vi "sys_get dynamic system class.vi"(11 "Dynamic System":T1) -> (2 "appended path":path, 3 "Dynamic-System out":refnum<class "Dynamic-System.lvclass">)   [LabVIEW 2025]
uses:
  Classes/Dynamic-System/Dynamic-System.lvclass
  Classes/mass-spring-damper/mass-spring-damper.lvclass
  Classes/water-tank/water-tank.lvclass
  C:/Users/grove/Desktop/LabVIEW/Git/dynamic-systems/Classes/Dynamic-System/Dynamic-System.lvclass
  C:/Users/grove/Desktop/LabVIEW/Git/dynamic-systems/Classes/mass-spring-damper/mass-spring-damper.lvclass
  C:/Users/grove/Desktop/LabVIEW/Git/dynamic-systems/Classes/water-tank/water-tank.lvclass
  Classes/Dynamic-System/dynamic system selection.ctl
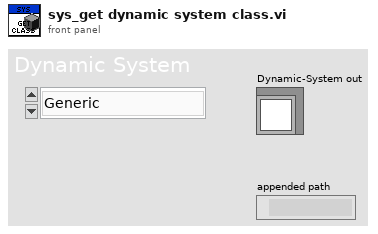
[diagram p1: front panel]
types:
  T1 = typedef "dynamic system selection.ctl" = enum16{"Generic", "Mass Spring Damper", "Water Tank", "RLC Circuit"}
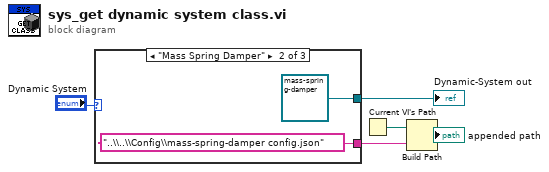
[diagram p0: block diagram]
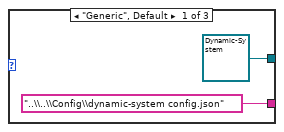
[diagram p2: hidden frame]
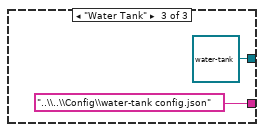
[diagram p3: hidden frame]
diagram:
  n1 = case shown="\"Mass Spring Damper\"" "Dynamic System" {
    tunnel: [refnum<class "Dynamic-System.lvclass"> refnum ("Dynamic-System.lvclass") refnum<class "mass-spring-damper.lvclass"> refnum ("mass-spring-damper.lvclass") refnum<class "water-tank.lvclass"> refnum ("water-tank.lvclass")] -> w2
    tunnel: ["..\\..\\Config\\dynamic-system config.json" "..\\..\\Config\\mass-spring-damper config.json" "..\\..\\Config\\water-tank config.json"] -> w4
    frame "Generic", Default {
    }
    frame "Mass Spring Damper" {
    }
    frame "Water Tank" {
    }
  }
  "Dynamic-System out" <- w2
  n2 = Current VI's Path() -> (path=w3:path)
  n3 = Build Path(base path=w3, name or relative path=w4) -> (appended path=→"appended path":path)
